vi "Shift Zero (single).vi"(8 "error in (no error)":errorcluster, 10 "Zero x index":i32, 11 "XY-data":cluster{"X-array":dbl[], "Y-array":dbl[]}) -> (0 "error out":errorcluster, 3 "Shifted XY-data out":cluster{"X-array":dbl[], "Y-array":dbl[]} {"Y-array" format="%.2p"; "X-array" format="%.2p"})   [LabVIEW 2019, in "xy_utilities.lvlib"]
doc: "Shift the zero value of the x array by giving a new fractional x index.\n\nWire data to the data input to determine the polymorphic instance to use or manually select the instance."
uses:
  xy_utilities.lvlib
  <vilib>/gmath/NI_Gmath.lvlib
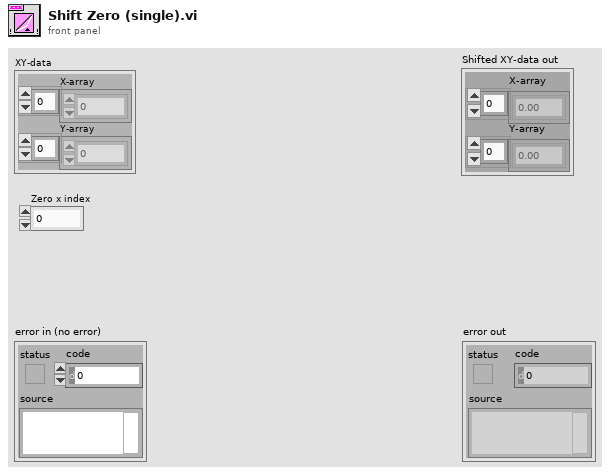
[diagram p1: front panel]
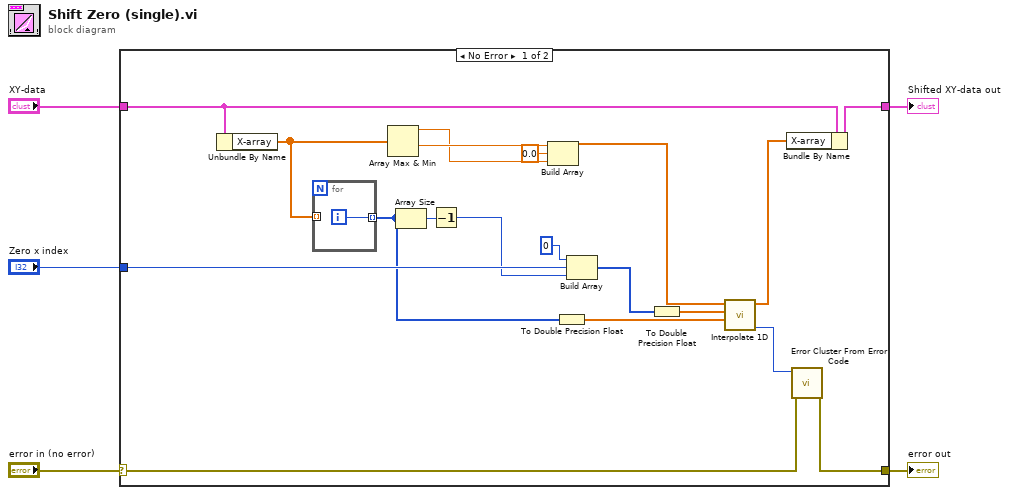
[diagram p0: block diagram]
diagram:
  n1 = case shown="No Error" "error in (no error)" {
    selector: "error in (no error)" -> [w6 w27]
    tunnel: [w10 w27] -> w4
    tunnel: "XY-data" -> [w7 w26]
    tunnel: [w24 w26] -> w2
    tunnel: "Zero x index" -> [w16 _]
    frame No Error {
      n2 = Unbundle By Name(w7) -> ("X-array"=w11:dbl[])
      n3 = for {
        tunnel: w11 -> [_] mode=indexing
        tunnel: [w25] -> w12 mode=indexing
        i -> [w25]
      }
      n4 = Array Max & Min(array=w11) -> (max value=w20:dbl, min value=w21:dbl)  [unwired: 2 out]
      n5 = Array Size(array=w12) -> (size(s)=w17:i32)
      n6 = Decrement(x=w17) -> (x-1=w15:i32)
      n7 = Build Array(w21, 0.0 ("element"), w20) -> (w13:dbl[])
      n8 = To Double Precision Float(number=w12) -> (double precision float=w8:dbl[])
      n9 = Build Array(0 ("element"), w16, w15) -> (w14:i32[])
      n10 = To Double Precision Float(number=w14) -> (double precision float=w9:dbl[])
      n11 = call <vilib>:"Interpolate 1D.vi"("xi"=w8, "X"=w9, "Y"=w13) -> ("error"=w23:i32, "yi"=w22:dbl[])  [unwired: 6 in, 1 out]
      n12 = Bundle By Name(cluster=w7, "X-array"=w22) -> (w24:cluster{"X-array":dbl[], "Y-array":dbl[]})
      n13 = call <vilib>:"Error Cluster From Error Code.vi"("error in (no error)"=w6, "error code (0)"=w23) -> ("error out"=w10:errorcluster)  [unwired: 7 in]
    }
    frame Error {
    }
  }
  "error out" <- w4
  "Shifted XY-data out" <- w2
